vi "3.4.vi"() -> ()   [LabVIEW 2019]
panel:
  out "Waveform Graph":u32[](graph)
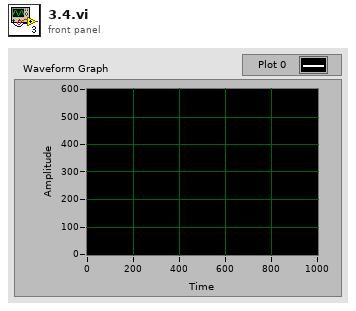
[diagram p1: front panel]
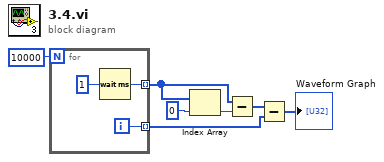
[diagram p0: block diagram]
diagram:
  n1 = for {
    N: 10000 -> [_]
    tunnel: [w9] -> w4 mode=indexing
    tunnel: [w8] -> w2 mode=indexing
    i -> [w8]
    n2 = Wait (ms)(milliseconds to wait=1) -> (millisecond timer value=w9:u32)
  }
  n3 = Index Array(array=w4, index=0) -> (element=w5:u32)
  n4 = Subtract(x=w4, y=w5) -> (x-y=w3:u32[])
  n5 = Subtract(x=w3, y=w2) -> (x-y=→"Waveform Graph":u32[])
